vi "Error Query.vi"(8 "error in (no error)":errorcluster, 11 "VISA resource name":refnum<visa-resource-name>) -> (0 "error out":errorcluster, 1 "Error Message":string, 2 "Error Code":i32, 3 "VISA resource name out":refnum<visa-resource-name>)   [LabVIEW 2014, in "GRBLMotionCore.lvlib"]
doc: "Queries the instrument for any errors in the instrument's error queue. It will continue to read errors until all errors have been read from the instrument. Any errors will be returned in the <B>error out</B> control.\n\n<B>Note:</B>\nThis VI is called automatically by most driver VIs so it is not usually necessary to call this in an application."
uses:
  <instrlib>/GRBL/GRBLMotionCore.lvlib
  <vilib>/regexp/Match Regular Expression.xnode
panel:
  # "EDIT: Note: The Error Query VI is included as a subVI in all driver VIs except low-level API VIs. If the instrument does not support error query, then remove the VI and remove subVI calls in each instrument driver VI that calls it."
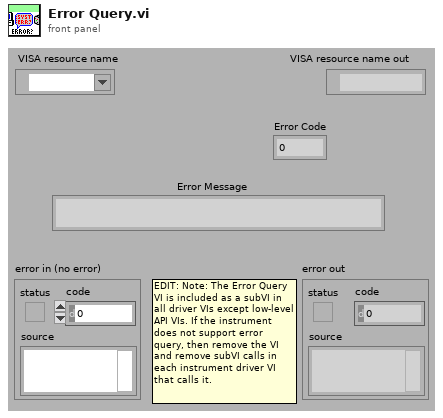
[diagram p1: front panel]
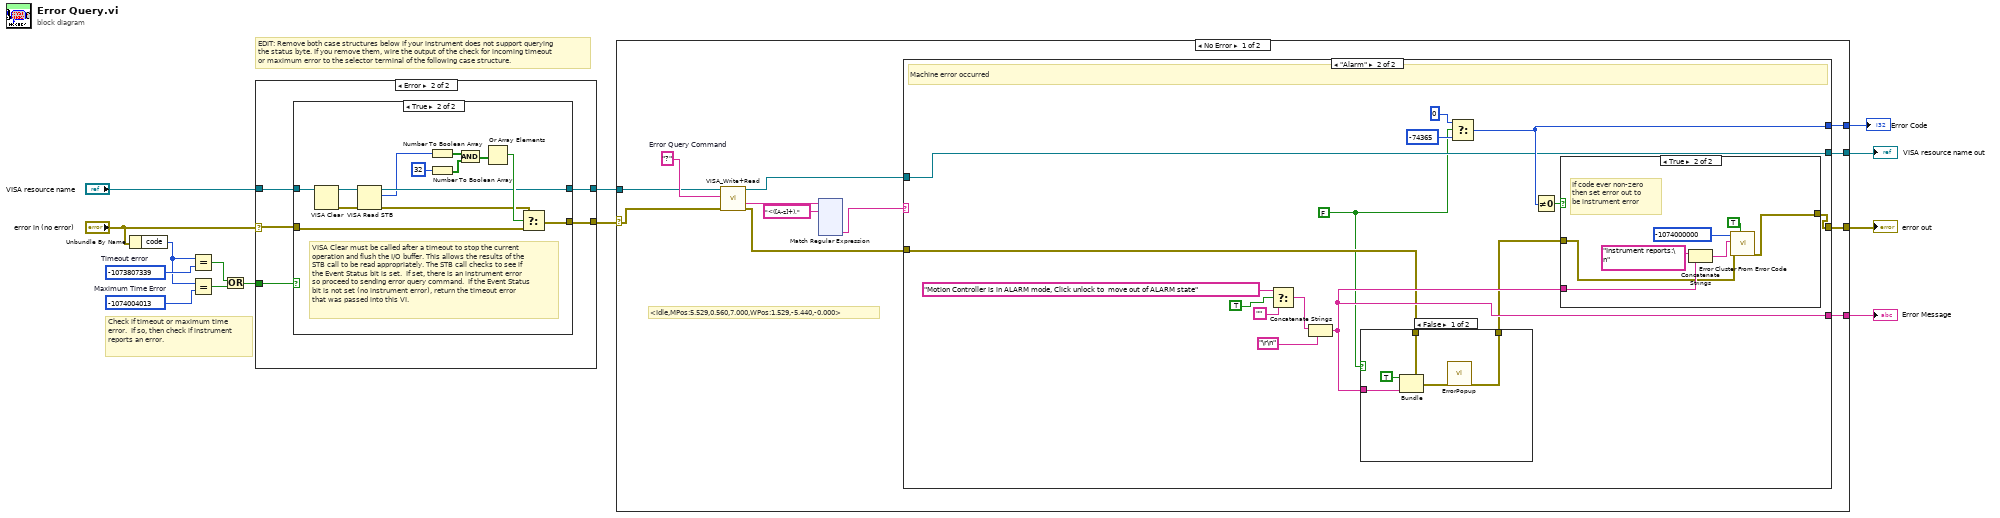
[diagram p0: block diagram]
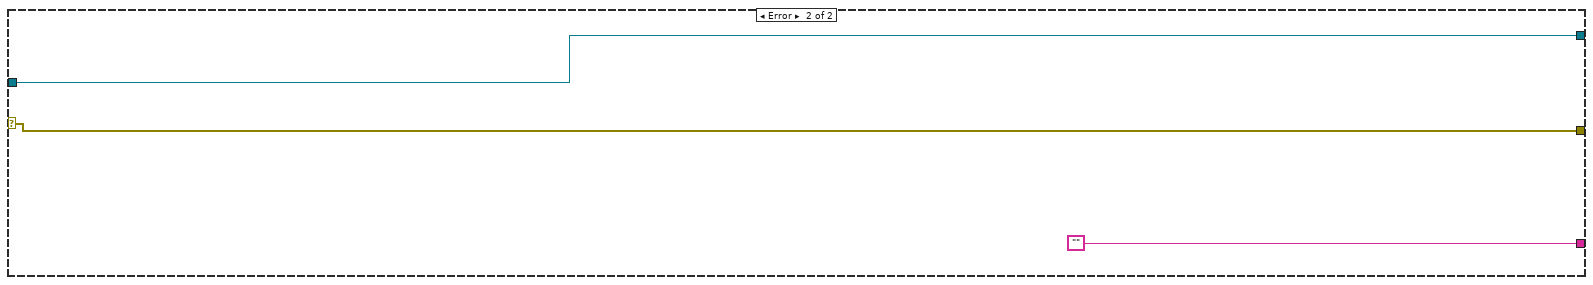
[diagram p7: hidden frame]
diagram:
  w6 = -1074004013  # Maximum Time Error
  w8 = -1073807339  # Timeout error
  # "Check if timeout or maximum time error.  If so, then check if instrument reports an error."
  # "EDIT: Remove both case structures below if your instrument does not support querying the status byte. If you remove them, wire the output of the check for incoming timeout or maximum error to the selector terminal of the following case structure."
  n1 = Unbundle By Name("error in (no error)") -> ("code"=w7:i32)
  n2 = Equal?(x=w7, y=w8) -> (x = y?=w4:bool)
  n3 = Equal?(x=w7, y=w6) -> (x = y?=w5:bool)
  n4 = Or(x=w4, y=w5) -> (x .or. y?=w3:bool)
  n5 = case shown="Error" "error in (no error)" {
    selector: "error in (no error)" -> [w15 w19]
    tunnel: "VISA resource name" -> [w16 w21]
    tunnel: [w16 w20] -> w10
    tunnel: [w15 w18] -> w11
    tunnel: w3 -> [_ w17]
    frame No Error {
    }
    frame Error {
      n6 = case shown="True" w17 {
        tunnel: w21 -> [w23 w29]
        tunnel: [w23 w26] -> w20
        tunnel: w19 -> [w22 w32]
        tunnel: [w22 w31] -> w18
        frame False {
          # "Error code not a timeout, so best to pass on to user."
        }
        frame True {
          # "VISA Clear must be called after a timeout to stop the current operation and flush the I/O buffer. This allows the results of the  STB call to be read appropriately. The STB call checks to see if the Event Status bit is set.  If set, there is an instrument error so proceed to sending error query command.  If the Event Status bit is not set (no instrument error), return the timeout error that was passed into this VI."
          n7 = VISA Clear(VISA resource name=w29) -> (VISA resource name out=w28:refnum<visa-resource-name>, error out=w27:errorcluster)  [unwired: 1 in]
          n8 = VISA Read STB(8:w27, 11:w28) -> (0:w25:errorcluster, 2:w24:u16, 3:w26:refnum<visa-resource-name>)
          n9 = Number To Boolean Array(number=w24) -> (Boolean array=w33:bool[])
          n10 = Number To Boolean Array(number=32) -> (Boolean array=w35:bool[])
          n11 = And(x=w33, y=w35) -> (x .and. y?=w34:bool[])
          n12 = Or Array Elements(Boolean array=w34) -> (logical OR=w30:bool)
          n13 = Select(t=w25, s=w30, f=w32) -> (s? t:f=w31:errorcluster)
        }
      }
    }
  }
  n14 = case shown="No Error" w11 {
    selector: w11 -> [w42 w196]
    tunnel: [w48 w198] -> w14
    tunnel: w10 -> [w43 w198]
    tunnel: [w47 w196] -> w13
    tunnel: [w46 ""] -> w12
    tunnel: [w45 _] -> w1
    frame No Error {
      w44 = "?"  # Error Query Command
      # "<Idle,MPos:5.529,0.560,7.000,WPos:1.529,-5.440,-0.000>"
      n15 = call <instrlib>:"VISA_Write+Read.vi"("error in (no error)"=w42, "Write Buffer"=w44, "VISA resource name"=w43) -> ("error out"=w41:errorcluster, "readout"=w39:string, "VISA resource name out"=w40:refnum<visa-resource-name>)  [unwired: 6 in]
      n16 = xnode "Match Regular Expression"("input string"=w39, "regular expression"="<([A-z]+),") -> ("submatch 1"=w37:string)  [unwired: 4 in, 5 out]
      n17 = case shown="\"Alarm\"" w37 {
        tunnel: [w165 w172] -> w48
        tunnel: [w166 w179] -> w47
        tunnel: [_ w178] -> w46
        tunnel: w41 -> [w166 w171]
        tunnel: w40 -> [w165 w172]
        tunnel: [_ w173] -> w45
        frame "False", Default {
        }
        frame "Alarm" {
          w168 = FALSE
          # "Machine error occurred"
          n18 = Select(t="Motion Controller is in ALARM mode, Click unlock to  move out of ALARM state", s=TRUE, f="") -> (s? t:f=w174:string)
          n19 = Concatenate Strings(w174, "\r\n") -> (w178:string)
          n20 = case shown="False" w168 {
            tunnel: w178 -> [w186 _]
            tunnel: w171 -> [w185 w187]
            tunnel: [w182 w187] -> w177
            frame False {
              n21 = Bundle(cluster=w185, "status"=TRUE, "source"=w186) -> (w183:errorcluster)  [unwired: 1 in]
              n22 = call <instrlib>:"ErrorPopup.vi"("error in (no error)"=w183) -> ("error out"=w182:errorcluster)  [unwired: 10 in]
            }
            frame True {
            }
          }
          n23 = Select(t=0, s=w168, f=-74365) -> (s? t:f=w173:i32)
          n24 = Not Equal To 0?(x=w173) -> (x != 0?=w180:bool)
          n25 = case shown="True" w180 {
            tunnel: w178 -> [_ w194]
            tunnel: [w188 w190] -> w179
            tunnel: w177 -> [w188 w189]
            frame False {
            }
            frame True {
              # "If code ever non-zero\nthen set error out to\nbe instrument error"
              n26 = Concatenate Strings("Instrument reports:\n" ("Source"), w194) -> (w191:string)
              n27 = call <vilib>:"Error Cluster From Error Code.vi"("show call chain? (False)"=TRUE, "error in (no error)"=w189, "error message (\"\")"=w191, "error code (0)"=-1074000000 ("Code")) -> ("error out"=w190:errorcluster)  [unwired: 5 in]
            }
          }
        }
      }
    }
    frame Error {
    }
  }
  "VISA resource name out" <- w14
  "error out" <- w13
  "Error Message" <- w12
  "Error Code" <- w1
